vi "REQ Broadcast DI.vi"(8 "error in":errorcluster, 10 "DI":bool[](array[boolean])) -> (0 "error out":errorcluster)   [LabVIEW 2016, in "DAQ Hardware.lvlib"]
doc: "_____\nCreated using DQMH Event Scripter 6.1.0.128."
uses:
  DAQ Hardware.lvlib
  REQ Broadcast DI Argument--cluster.ctl
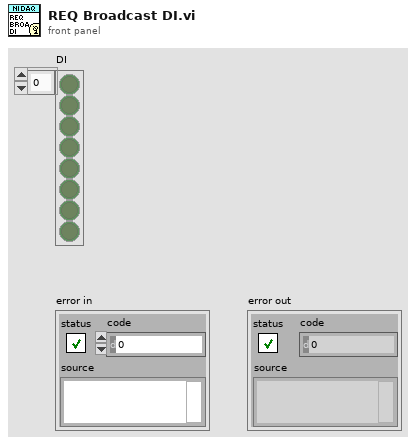
[diagram p1: front panel]
types:
  T1 = typedef "DAQ Hardware.lvlib/REQ Broadcast DI Argument--cluster.ctl" = cluster{"DI":bool[]}
  T2 = typedef "DAQ Hardware.lvlib/Broadcast Events--cluster.ctl" = cluster{"Module Did Init":refnum<user-event>, "Status Updated":refnum<user-event>, "Error Reported":refnum<user-event>, "Module Did Stop":refnum<user-event>, "Update Module Execution Status":refnum<user-event>, "REQ Broadcast DI":refnum<user-event>, "REQ Broad AI":refnum<user-event>}
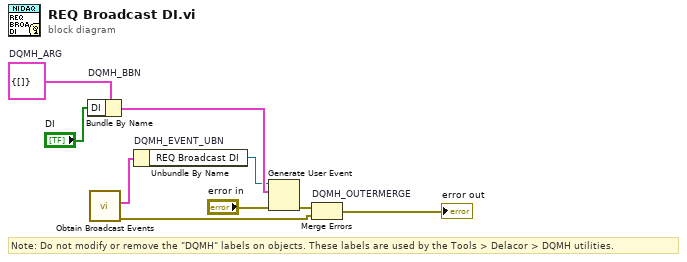
[diagram p0: block diagram]
diagram:
  w4 = T1 {"DI"=[]}  # DQMH_ARG
  # "Note: Do not modify or remove the \"DQMH\" labels on objects. These labels are used by the Tools > Delacor > DQMH utilities."
  n1 = Bundle By Name "DQMH_BBN"(cluster=w4, "DI"="DI") -> (w7:T1)
  n2 = call "Obtain Broadcast Events.vi"() -> ("error out"=w2:errorcluster, "DAQ Hardware Broadcast Events"=w1:T2)  [unwired: 10 in]
  n3 = Unbundle By Name "DQMH_EVENT_UBN"(w1) -> ("REQ Broadcast DI"=w6:refnum<user-event>)
  n4 = Generate User Event(user event=w6, event data cluster=w7, error in="error in") -> (error out=w5:errorcluster)  [unwired: 1 in, 1 out]
  n5 = Merge Errors "DQMH_OUTERMERGE"(w5, w2) -> (→"error out":errorcluster)
